vi "Build Bundle Display Name.vi"(10 "Nest Chain":string[](array[string]), 11 "Element Label":string) -> (3 "Bundle display name":string)   [LabVIEW 2023]
doc: "Build bundle display name from nest chain and element label\n\nElement Label = '\"C\"\nNest Chain = [\"A\",\"B\"]\n\ndisplay name = \"A.B.C\"\n\nThis is how the name will appear in a named bundler, and must be exact."
uses:
  <vilib>/Utility/error.llb/Trim Whitespace One-Sided.vi
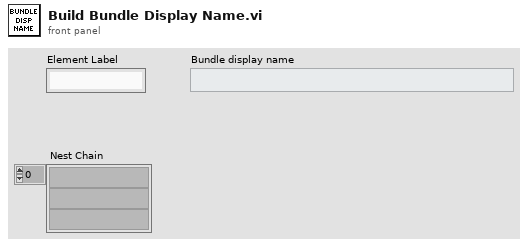
[diagram p1: front panel]
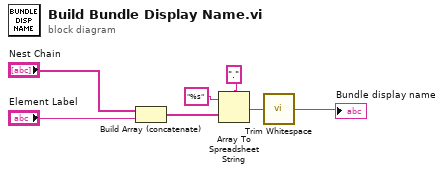
[diagram p0: block diagram]
diagram:
  n1 = Build Array (concatenate)("Nest Chain", "Element Label") -> (w2:string[])
  n2 = Array To Spreadsheet String(delimiter (Tab)=".", array=w2, 3:"%s" ("format string")) -> (spreadsheet string=w6:string)
  n3 = call <vilib>:"Trim Whitespace.vi"("string"=w6) -> ("trimmed string"=→"Bundle display name":string)  [unwired: 1 in]
